vi "set_internal_files.vi"(8 "error in (no error)":errorcluster, 11 "device_type in":refnum<class "device_type.lvclass">) -> (0 "error out":errorcluster, 3 "device_type out":refnum<class "device_type.lvclass">)   [LabVIEW 2021, in "device_type.lvclass"]
uses:
  device_type.lvclass
  device_type.lvclass/device_type.ctl
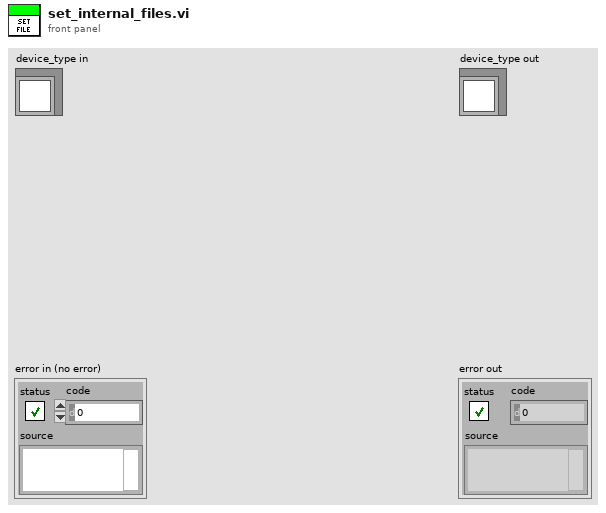
[diagram p1: front panel]
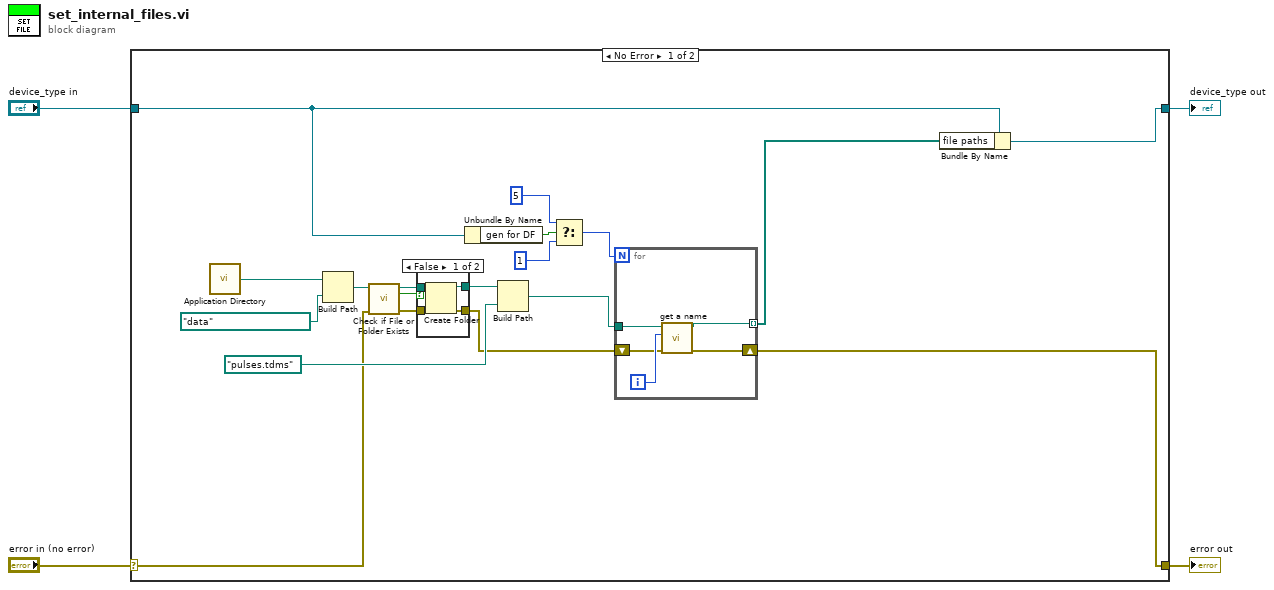
[diagram p0: block diagram]
diagram:
  n1 = case shown="No Error" "error in (no error)" {
    selector: "error in (no error)" -> [w7 w36]
    tunnel: [w23 w36] -> w3
    tunnel: [w18 w35] -> w1
    tunnel: "device_type in" -> [w17 w35]
    frame No Error {
      n2 = call <vilib>:"Application Directory.vi"() -> ("Application Directory"=w14:path)
      n3 = Build Path(base path=w14, name or relative path=path "data") -> (appended path=w11:path)
      n4 = call <vilib>:"Check if File or Folder Exists.vi"("error in (no error)"=w7, "path"=w11) -> ("error out"=w8:errorcluster, "file or folder exists?"=w5:bool, "dup path"=w10:path)  [unwired: 7 in]
      n5 = case shown="False" w5 {
        tunnel: w10 -> [w27 w29]
        tunnel: [w26 w29] -> w9
        tunnel: w8 -> [w25 w28]
        tunnel: [w24 w28] -> w6
        frame False {
          n6 = Create Folder(path (use dialog)=w27, error in=w25) -> (created path=w26:path, error out=w24:errorcluster)  [unwired: 1 in, 1 out]
        }
        frame True {
        }
      }
      n7 = Unbundle By Name(w17) -> ("gen for DF"=w21:bool)
      n8 = Build Path(base path=w9, name or relative path=path "pulses.tdms") -> (appended path=w12:path)
      n9 = Select(t=5, s=w21, f=1) -> (s? t:f=w22:i32)
      n10 = for {
        N: w22 -> [_]
        tunnel: w12 -> [w34]
        shift-right: [w31] -> w23
        shift-left: w6 -> [w32]
        tunnel: [w30] -> w16 mode=indexing
        i -> [w33]
        n11 = call "get a name.vi"("error constant"=w32, "Numeric"=w33, "Bitfile path"=w34) -> ("error constant 2"=w31:errorcluster, "Path"=w30:path)  [unwired: 7 in]
      }
      n12 = Bundle By Name(cluster=w17, "file paths"=w16) -> (w18:refnum<class "device_type.lvclass">)
    }
    frame Error {
    }
  }
  "error out" <- w3
  "device_type out" <- w1
